vi "SubVI_THD.vi"(10 "Osciloscópio":refnum<visa-resource-name>="GPIB0::1::INSTR") -> (2 "THD":dbl format="%.2p", 3 "VISA resource name out":refnum<visa-resource-name>)   [LabVIEW 2021]
uses:
  Agilent 6000 Series/Public/Data/Read Single Waveform.vi
  <vilib>/measure/matone.llb/Harmonic Distortion Analyzer 1 Chan.vi
  <vilib>/measure/NI_MAPro.lvlib
  Agilent 6000 Series/Agilent 6000 Series.lvlib
panel:
  out "Waveform Graph":waveform(dbl)(graph)
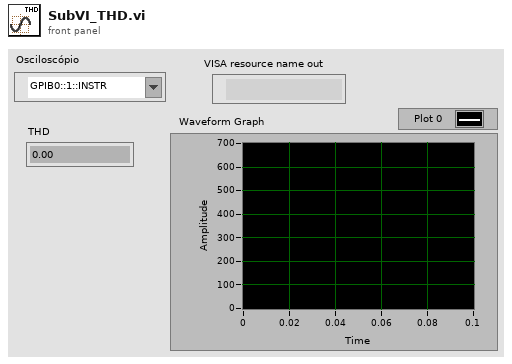
[diagram p1: front panel]
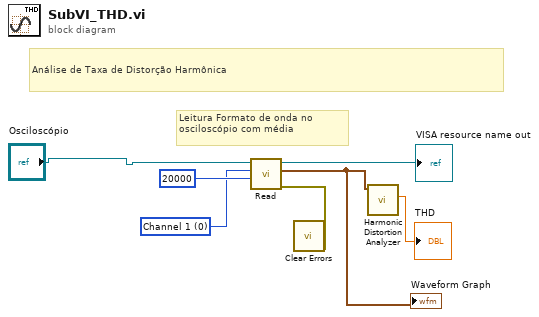
[diagram p0: block diagram]
diagram:
  w3 = u16 0 items=["Channel 1", "Channel 2", "Channel 3", "Channel 4", "Math"] ("Source (0: Channel 1)")
  # "Análise de Taxa de Distorção Harmônica"
  # "Leitura Formato de onda no \nosciloscópio com média"
  n1 = call-poly "Read.vi"("Timeout (10000 ms)"=u32 20000, "Source (0: Channel 1)"=w3, "VISA resource name"="Osciloscópio") -> ("error out"=w5:errorcluster, "Waveform Data"=w2:waveform(dbl), "VISA resource name out"=→"VISA resource name out":refnum<visa-resource-name>)  [unwired: 6 in]
  "Waveform Graph" <- w2
  n2 = call <vilib>:"Clear Errors.vi"("error in (no error)"=w5) -> ()  [unwired: 5 in, 2 out]
  n3 = call-poly <vilib>:"Harmonic Distortion Analyzer.vi"("signal in"=w2) -> ("THD"=→"THD":dbl)  [unwired: 5 in, 5 out]
